vi "Topological Sort.vi"(8 "error in (no error)":errorcluster, 11 "Topological Sort in":refnum<class "Topological Sort.lvclass">) -> (0 "error out":errorcluster, 3 "Topological Sort out":refnum<class "Topological Sort.lvclass">)   [LabVIEW 2025, in "AOC.lvlib" / "Topological Sort.lvlib" / "Topological Sort.lvclass"]
uses:
  Topological Sort.lvclass
  Topological Sort.lvclass/Topological Sort.ctl
  Graph/Graph.lvclass
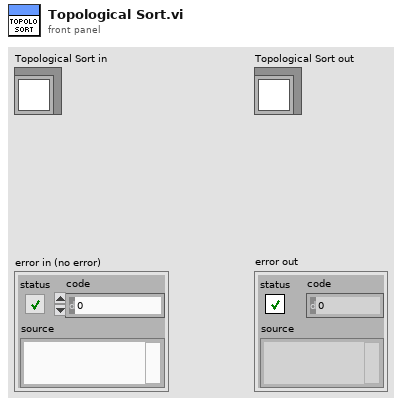
[diagram p1: front panel]
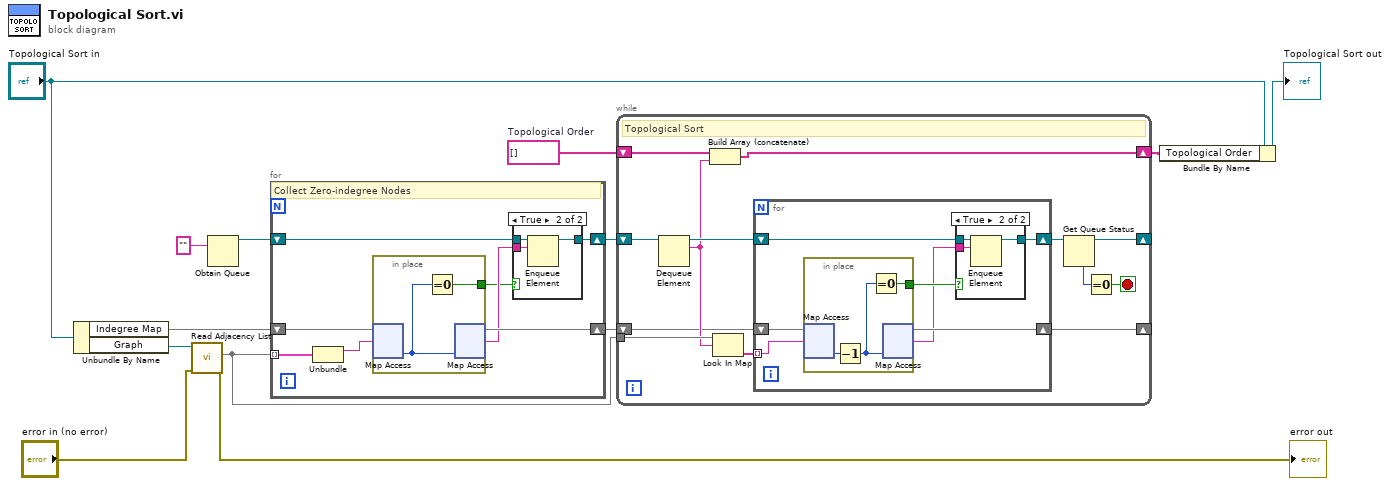
[diagram p0: block diagram]
diagram:
  w12 = string[] []  # Topological Order
  n1 = Unbundle By Name("Topological Sort in") -> ("Indegree Map"=w7:map{string, u64}, "Graph"=w6:refnum<class "Graph.lvclass">)
  n2 = call-dynamic "Read Adjacency List.vi"("error in (no error)"="error in (no error)", "Graph in"=w6) -> ("error out"=→"error out":errorcluster, "Adjacency List"=w5:map{string, string[]})  [unwired: 7 in, 1 out]
  n3 = Obtain Queue(element data type="") -> (queue out=w10:refnum<queue>)  [unwired: 4 in, 2 out]
  n4 = for {
    tunnel: w5 -> [w19] mode=indexing
    shift-right: [w20] -> w13
    shift-left: w7 -> [w21]
    shift-right: [w17] -> w11
    shift-left: w10 -> [w18]
    # "Collect Zero-indegree Nodes"
    n5 = Unbundle(w19) -> (w14:string)  [unwired: 1 out]
    n6 = in-place {
      in-place-border: [w26] -> w15
      n7 = in-place-map #1(w21, w14) -> (w27:u64)  [unwired: 1 in, 1 out]
      n8 = Equal To 0?(x=w27) -> (x = 0?=w26:bool)
      n9 = in-place-map #1(w27) -> (w20:map{string, u64}, w16:string)  [unwired: 1 in, 1 out]
    }
    n10 = case shown="True" w15 {
      tunnel: w18 -> [w22 w25]
      tunnel: [w22 w24] -> w17
      tunnel: w16 -> [_ w23]
      frame False {
      }
      frame True {
        n11 = Enqueue Element(queue=w25, element=w23) -> (queue out=w24:refnum<queue>)  [unwired: 2 in, 2 out]
      }
    }
  }
  n12 = while {
    tunnel: w5 -> [w39]
    shift-right: [w35] -> _
    shift-left: w11 -> [w40]
    shift-right: [w29] -> _
    shift-left: w13 -> [w30]
    shift-right: [w28] -> w1
    shift-left: w12 -> [w32]
    stop <- w33 stop-if-true
    # "Topological Sort"
    n13 = Dequeue Element(queue=w40) -> (queue out=w37:refnum<queue>, element=w31:string)  [unwired: 2 in, 2 out]
    n14 = Build Array (concatenate)(w32, w31) -> (w28:string[])
    n15 = Look In Map(map=w39, key=w31) -> (value=w38:string[])  [unwired: 1 in, 1 out]
    n16 = for {
      tunnel: w38 -> [w46] mode=indexing
      shift-right: [w41] -> w36
      shift-left: w37 -> [w44]
      shift-right: [w45] -> w29
      shift-left: w30 -> [w47]
      n17 = in-place {
        in-place-border: [w52] -> w43
        n18 = in-place-map #2(w47, w46) -> (w54:u64)  [unwired: 1 in, 1 out]
        n19 = Decrement(x=w54) -> (x-1=w53:u64)
        n20 = Equal To 0?(x=w53) -> (x = 0?=w52:bool)
        n21 = in-place-map #2(w53) -> (w45:map{string, u64}, w42:string)  [unwired: 1 in, 1 out]
      }
      n22 = case shown="True" w43 {
        tunnel: w44 -> [w48 w51]
        tunnel: [w48 w50] -> w41
        tunnel: w42 -> [_ w49]
        frame False {
        }
        frame True {
          n23 = Enqueue Element(queue=w51, element=w49) -> (queue out=w50:refnum<queue>)  [unwired: 2 in, 2 out]
        }
      }
    }
    n24 = Get Queue Status(queue=w36) -> (queue out=w35:refnum<queue>, # elements in queue=w34:i32)  [unwired: 2 in, 6 out]
    n25 = Equal To 0?(x=w34) -> (x = 0?=w33:bool)
  }
  n26 = Bundle By Name(cluster="Topological Sort in", "Topological Order"=w1) -> (→"Topological Sort out":refnum<class "Topological Sort.lvclass">)
